vi "Is Open Delimiter.vi"(8 "Error In":errorcluster, 11 "Lexer In":refnum<class "Lexer.lvclass">) -> (0 "Error Out":errorcluster, 2 "Open Delimiter":bool, 3 "Lexer Out":refnum<class "Lexer.lvclass">)   [LabVIEW 2018, in "Toolkit.lvlib" / "Lexer.lvclass"]
uses:
  Lexer.lvclass
  Lexer.lvclass/Lexer.ctl
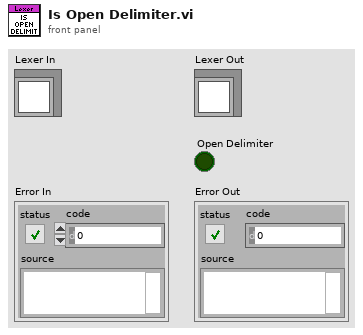
[diagram p1: front panel]
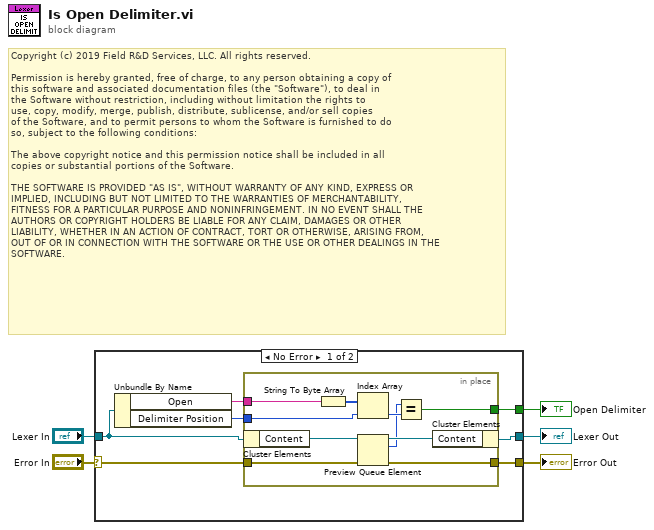
[diagram p0: block diagram]
diagram:
  # "Copyright (c) 2019 Field R&D Services, LLC. All rights reserved.\n\nPermission is hereby granted, free of charge, to any person obtaining a copy of\nthis software and associated documentation files (the \"Software\"), to deal in\nthe Software without restriction, including without limitation the rights to\nuse, copy, modify, merge, publish, distribute, sublicense, and/or sell copies\nof the Software, and to permit persons to whom the Software is furnished to do\nso, subject to the following conditions:\n\nThe above copyright notice and this permission notice shall be included in all\ncopies or substantial portions of the Software.\n\nTHE SOFTWARE IS PROVIDED \"AS IS\", WITHOUT WARRANTY OF ANY KIND, EXPRESS OR\nIMPLIED, INCLUDING BUT NOT LIMITED TO THE WARRANTIES OF MERCHANTABILITY,\nFITNESS FOR A PARTICULAR PURPOSE AND NONINFRINGEMENT. IN NO EVENT SHALL THE\nAUTHORS OR COPYRIGHT HOLDERS BE LIABLE FOR ANY CLAIM, DAMAGES OR OTHER\nLIABILITY, WHETHER IN AN ACTION OF CONTRACT, TORT OR OTHERWISE, ARISING FROM,\nOUT OF OR IN CONNECTION WITH THE SOFTWARE OR THE USE OR OTHER DEALINGS IN THE\nSOFTWARE."
  n1 = case shown="No Error" "Error In" {
    selector: "Error In" -> [w7 w24]
    tunnel: [w6 w24] -> w4
    tunnel: "Lexer In" -> [w12 w23]
    tunnel: [w11 w23] -> w2
    tunnel: [w8 _] -> w1
    frame No Error {
      n2 = Unbundle By Name(w12) -> ("Open"=w9:string, "Delimiter Position"=w10:i32)
      n3 = in-place {
        in-place-border: w10 -> [w20]
        in-place-border: w9 -> [w19]
        in-place-border: [w18] -> w8
        in-place-border: w7 -> [w14]
        in-place-border: [w13] -> w6
        n4 = in-place-cluster #1(w12) -> ("Content"=w17:refnum<queue>)
        n5 = String To Byte Array(string=w19) -> (unsigned byte array=w21:u8[])
        n6 = Index Array(array=w21, index=w20) -> (element=w22:u8)
        n7 = Preview Queue Element(queue=w17, error in (no error)=w14) -> (queue out=w16:refnum<queue>, element=w15:u8, error out=w13:errorcluster)  [unwired: 1 in, 1 out]
        n8 = Equal?(x=w15, y=w22) -> (x = y?=w18:bool)
        n9 = in-place-cluster #1("Content"=w16) -> (w11:refnum<class "Lexer.lvclass">)
      }
    }
    frame Error {
    }
  }
  "Error Out" <- w4
  "Lexer Out" <- w2
  "Open Delimiter" <- w1
